vi "Waveform Graph.vi"() -> ()   [LabVIEW 2021]
panel:
  out "Temp + Sin":dbl[][](graph)
  out "Sin":dbl[](graph)
  out "Temp":dbl[](array[numeric])
  out "Temp + Scale":cluster{i32, i32, dbl[]}(graph)
  in  "Temp Scale":bool
  in  "Knob":dbl(knob) scale=0.0..100.0
  out "Temp":dbl[](graph)
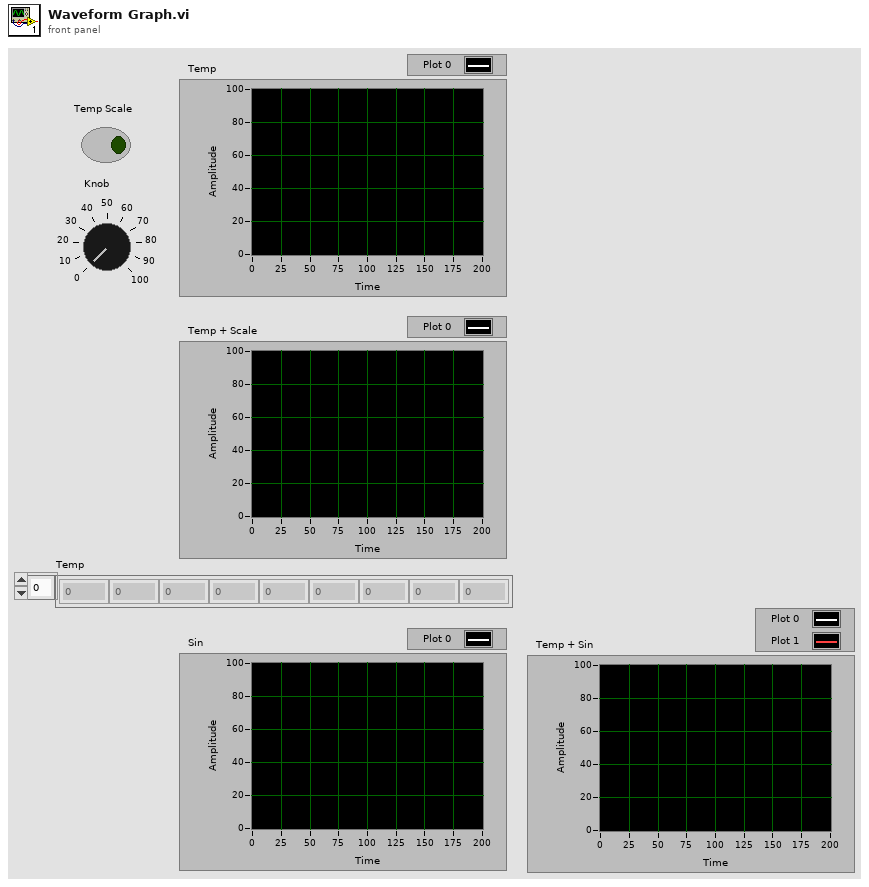
[diagram p1: front panel]
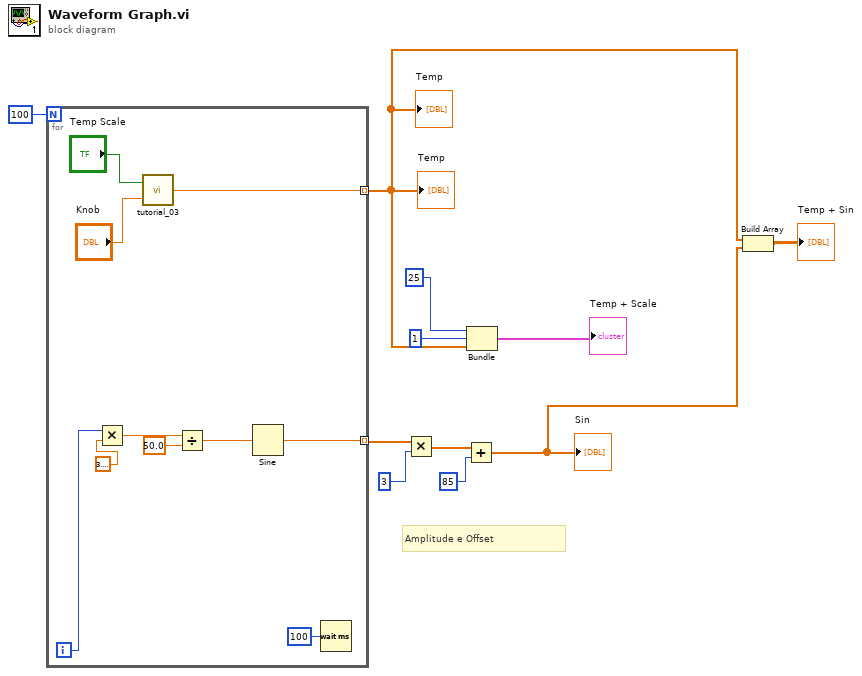
[diagram p0: block diagram]
diagram:
  # "Amplitude e Offset"
  n1 = for {
    N: 100 -> [_]
    tunnel: [w21] -> w2 mode=indexing
    tunnel: [w12] -> w6 mode=indexing
    i -> [w14]
    n2 = Multiply(x=w14, y=3.141592653589793) -> (x*y=w16:dbl)
    n3 = call "tutorial_03.vi"("Knob"="Knob", "Temp Scale"="Temp Scale") -> ("Thermometer"=w21:dbl)
    n4 = Divide(x=w16, y=50.0) -> (x/y=w17:dbl)
    n5 = Sine(x=w17) -> (sin(x)=w12:dbl)
    n6 = Wait (ms)(milliseconds to wait=u32 100) -> ()  [unwired: 1 out]
  }
  "Temp" <- w2
  "Temp" <- w2
  n7 = Multiply(x=w6, y=3) -> (x*y=w7:dbl[])
  n8 = Add(x=w7, y=85) -> (x+y=w1:dbl[])
  "Sin" <- w1
  n9 = Bundle(25, 1, w2) -> (→"Temp + Scale":cluster{i32, i32, dbl[]})  [unwired: 1 in]
  n10 = Build Array(w2, w1) -> (→"Temp + Sin":dbl[][])
